vi "Signal Routing.vi"(10 "Boolean Array":bool[](array[boolean]), 11 "Data In":dynamicdata[](array[waveform])) -> (3 "Output":T1)   [LabVIEW 2022 SP3]
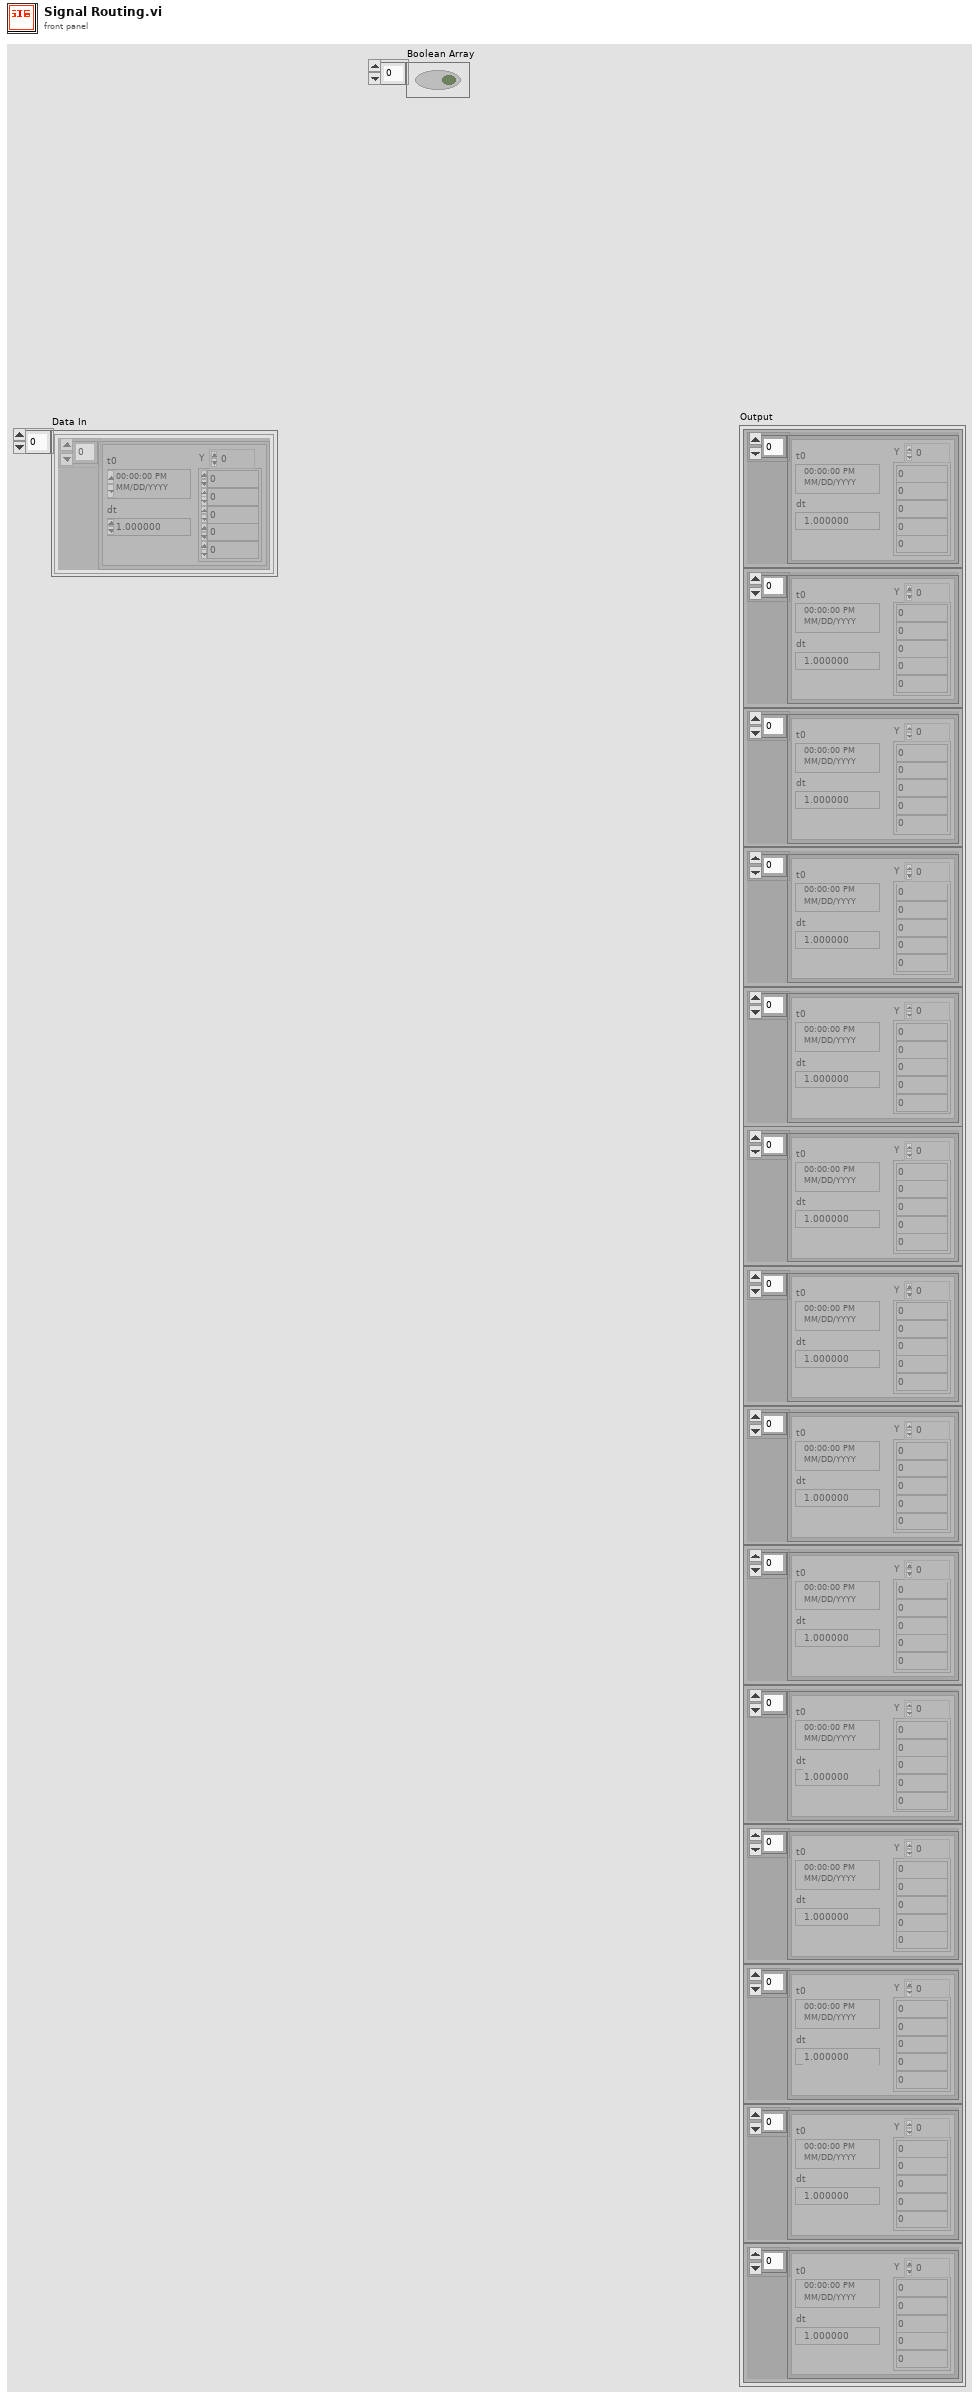
[diagram p1: front panel]
types:
  T1 = cluster{"Dynamic Data":dynamicdata, "Dynamic Data":dynamicdata, "Dynamic Data":dynamicdata, "Dynamic Data":dynamicdata, "Dynamic Data":dynamicdata, "Dynamic Data":dynamicdata, "Dynamic Data":dynamicdata, "Dynamic Data":dynamicdata, "Dynamic Data":dynamicdata, "Dynamic Data":dynamicdata, "Dynamic Data":dynamicdata, "Dynamic Data":dynamicdata, "Dynamic Data":dynamicdata, "Dynamic Data":dynamicdata}
  T2 = cluster{dynamicdata, dynamicdata, dynamicdata, dynamicdata, dynamicdata, dynamicdata, dynamicdata, dynamicdata, dynamicdata, dynamicdata, dynamicdata, dynamicdata, dynamicdata, dynamicdata}
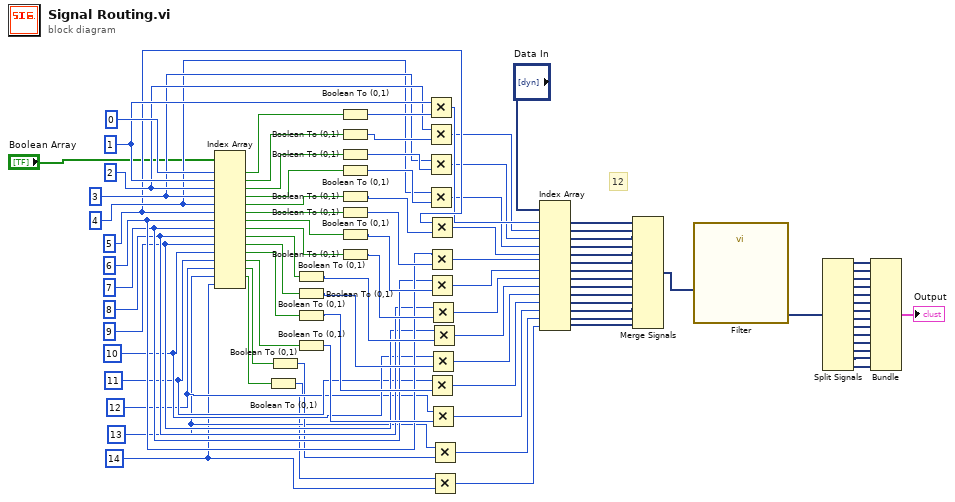
[diagram p0: block diagram]
diagram:
  w7 = 14 ("index")
  w11 = 13 ("index")
  w42 = 12 ("index")
  w43 = 11 ("index")
  w44 = 10 ("index")
  w45 = 9 ("index")
  w58 = 8 ("index")
  w59 = 7 ("index")
  w60 = 6 ("index")
  w61 = 5 ("index")
  w62 = 4 ("index")
  w63 = 3 ("index")
  w64 = 2 ("index")
  w65 = 1 ("index")
  # "12"
  n1 = Index Array(array="Boolean Array", index #1=0 ("index"), index #2=w65, index #3=w64, index #4=w63, index #5=w62, index #6=w61, index #7=w60, index #8=w59, index #9=w58, index #10=w45, index #11=w44, index #12=w43, index #13=w42, index #14=w11, index #15=w7) -> (element #1=w89:bool, element #2=w88:bool, element #3=w87:bool, element #4=w86:bool, element #5=w85:bool, element #6=w84:bool, element #7=w83:bool, element #8=w82:bool, element #9=w81:bool, element #10=w80:bool, element #11=w79:bool, element #12=w78:bool, element #13=w13:bool, element #14=w9:bool)  [unwired: 1 out]
  n2 = Boolean To (0,1)(Boolean=w9) -> (0, 1=w8:i16)
  n3 = Boolean To (0,1)(Boolean=w13) -> (0, 1=w12:i16)
  n4 = Boolean To (0,1)(Boolean=w81) -> (0, 1=w69:i16)
  n5 = Boolean To (0,1)(Boolean=w80) -> (0, 1=w68:i16)
  n6 = Boolean To (0,1)(Boolean=w79) -> (0, 1=w67:i16)
  n7 = Boolean To (0,1)(Boolean=w78) -> (0, 1=w66:i16)
  n8 = Boolean To (0,1)(Boolean=w89) -> (0, 1=w77:i16)
  n9 = Boolean To (0,1)(Boolean=w88) -> (0, 1=w76:i16)
  n10 = Boolean To (0,1)(Boolean=w87) -> (0, 1=w75:i16)
  n11 = Boolean To (0,1)(Boolean=w86) -> (0, 1=w74:i16)
  n12 = Boolean To (0,1)(Boolean=w85) -> (0, 1=w73:i16)
  n13 = Boolean To (0,1)(Boolean=w84) -> (0, 1=w72:i16)
  n14 = Boolean To (0,1)(Boolean=w83) -> (0, 1=w71:i16)
  n15 = Boolean To (0,1)(Boolean=w82) -> (0, 1=w70:i16)
  n16 = Multiply(x=w65, y=w77) -> (x*y=w57:i32)
  n17 = Multiply(x=w64, y=w76) -> (x*y=w56:i32)
  n18 = Multiply(x=w63, y=w75) -> (x*y=w55:i32)
  n19 = Multiply(x=w62, y=w74) -> (x*y=w54:i32)
  n20 = Multiply(x=w61, y=w73) -> (x*y=w53:i32)
  n21 = Multiply(x=w60, y=w72) -> (x*y=w52:i32)
  n22 = Multiply(x=w59, y=w71) -> (x*y=w51:i32)
  n23 = Multiply(x=w43, y=w67) -> (x*y=w47:i32)
  n24 = Multiply(x=w58, y=w70) -> (x*y=w50:i32)
  n25 = Multiply(x=w44, y=w68) -> (x*y=w48:i32)
  n26 = Multiply(x=w42, y=w66) -> (x*y=w46:i32)
  n27 = Multiply(x=w45, y=w69) -> (x*y=w49:i32)
  n28 = Multiply(x=w11, y=w12) -> (x*y=w10:i32)
  n29 = Multiply(x=w8, y=w7) -> (x*y=w6:i32)
  n30 = Index Array(array="Data In", index #1=w57, index #2=w56, index #3=w55, index #4=w54, index #5=w53, index #6=w52, index #7=w51, index #8=w50, index #9=w49, index #10=w48, index #11=w47, index #12=w46, index #13=w10, index #14=w6) -> (element #1=w28:dynamicdata, element #2=w29:dynamicdata, element #3=w30:dynamicdata, element #4=w31:dynamicdata, element #5=w32:dynamicdata, element #6=w33:dynamicdata, element #7=w34:dynamicdata, element #8=w35:dynamicdata, element #9=w36:dynamicdata, element #10=w37:dynamicdata, element #11=w38:dynamicdata, element #12=w39:dynamicdata, element #13=w5:dynamicdata, element #14=w4:dynamicdata)
  n31 = Merge Signals(w28, w29, w30, w31, w32, w33, w34, w35, w36, w37, w38, w39, w5, w4) -> (w27:dynamicdata)
  n32 = call "Filter"("Signal"=w27) -> ("Filtered Signal"=w26:dynamicdata)  [unwired: 9 in, 1 out]
  n33 = Split Signals(w26) -> (w25:dynamicdata, w24:dynamicdata, w23:dynamicdata, w22:dynamicdata, w21:dynamicdata, w20:dynamicdata, w19:dynamicdata, w18:dynamicdata, w17:dynamicdata, w16:dynamicdata, w14:dynamicdata, w15:dynamicdata, w3:dynamicdata, w2:dynamicdata)  [unwired: 14 in]
  n34 = Bundle(w25, w24, w23, w22, w21, w20, w19, w18, w17, w16, w14, w15, w3, w2) -> (→"Output":T2)  [unwired: 1 in]
